vi "BRig_dataTrial_DAB_I_HighProbSel.vi"() -> (2 "output_DAB_I_HighProbSel":i32)   [LabVIEW 2014]
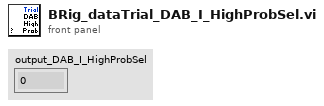
[diagram p1: front panel]
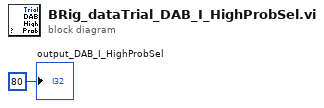
[diagram p0: block diagram]
diagram:
  "output_DAB_I_HighProbSel" <- 80 ("output_iBlock")
